vi "Channel DAQ.vi"() -> ()   [LabVIEW 2025]
uses:
  <vilib>/DAQmx/write.llb/DAQmx Write (Digital Bool 1Line 1Point).vi
  <vilib>/DAQmx/read.llb/DAQmx Read (Digital Bool 1Line 1Point).vi
  <vilib>/DAQmx/create/channels.llb/DAQmx Create Channel (DO-Digital Output).vi
  <vilib>/DAQmx/create/channels.llb/DAQmx Create Channel (DI-Digital Input).vi
  <vilib>/DAQmx/miscellaneous.llb/DAQmx Fill In Error Info.vi
panel:
  in  "Stop":bool
  in  "Write":bool
  out "Read":bool
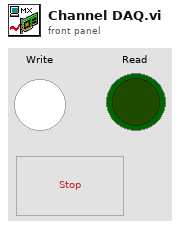
[diagram p1: front panel]
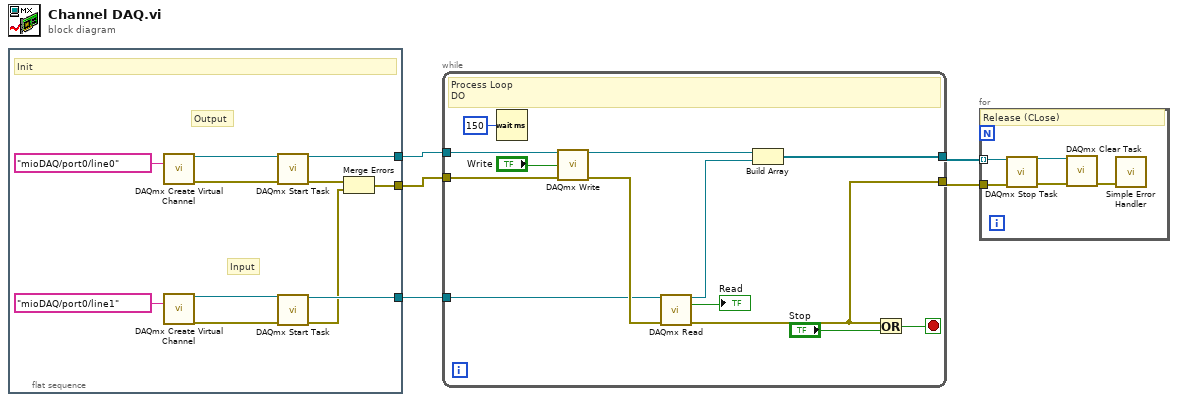
[diagram p0: block diagram]
diagram:
  n1 = flat-sequence {
    tunnel: [w16] -> w5
    tunnel: [w14] -> w2
    tunnel: [w13] -> w1
    frame #0 {
      # "Input"
      # "Output"
      # "Init"
      n2 = call-poly <vilib>:"DAQmx Create Virtual Channel.vi"("lines"=tag "mioDAQ/port0/line0") -> ("task out"=w11:refnum<k21>, "error out"=w10:errorcluster)  [unwired: 13 in]
      n3 = call-poly <vilib>:"DAQmx Create Virtual Channel.vi"("lines"=tag "mioDAQ/port0/line1") -> ("task out"=w7:refnum<k21>, "error out"=w6:errorcluster)  [unwired: 13 in]
      n4 = call <vilib>:"DAQmx Start Task.vi"("task/channels in"=w11, "error in"=w10) -> ("task out"=w16:refnum<k21>, "error out"=w15:errorcluster)  [unwired: 12 in]
      n5 = call <vilib>:"DAQmx Start Task.vi"("task/channels in"=w7, "error in"=w6) -> ("task out"=w14:refnum<k21>, "error out"=w12:errorcluster)  [unwired: 12 in]
      n6 = Merge Errors(w15, w12) -> (w13:errorcluster)
    }
  }
  n7 = while {
    tunnel: w5 -> [w29]
    tunnel: w1 -> [w27]
    tunnel: [w18] -> w4
    tunnel: [w21] -> w3
    tunnel: w2 -> [w20]
    stop <- w23 stop-if-true
    # "Process Loop\nDO"
    n8 = Wait (ms)(milliseconds to wait=u32 150) -> ()  [unwired: 1 out]
    n9 = call-poly <vilib>:"DAQmx Write.vi"("task/channels in"=w29, "data"="Write", "error in"=w27) -> ("task out"=w25:refnum<k21>, "error out"=w22:errorcluster)  [unwired: 10 in, 1 out]
    n10 = call-poly <vilib>:"DAQmx Read.vi"("task/channels in"=w20, "error in"=w22) -> ("task out"=w17:refnum<k21>, "data"=→"Read":bool, "error out"=w21:errorcluster)  [unwired: 11 in]
    n11 = Build Array(w25, w17) -> (w18:refnum<k21>[])
    n12 = Or(x=w21, y="Stop") -> (x .or. y?=w23:bool)
  }
  n13 = for {
    tunnel: w4 -> [w34] mode=indexing
    tunnel: w3 -> [w33]
    # "Release (CLose)"
    n14 = call <vilib>:"DAQmx Stop Task.vi"("task/channels in"=w34, "error in"=w33) -> ("task out"=w31:refnum<k21>, "error out"=w32:errorcluster)  [unwired: 12 in]
    n15 = call <vilib>:"DAQmx Clear Task.vi"("task in"=w31, "error in"=w32) -> ("error out"=w30:errorcluster)  [unwired: 13 in]
    n16 = call <vilib>:"Simple Error Handler.vi"("error in (no error)"=w30) -> ()  [unwired: 4 in, 5 out]
  }
